vi "UHR-Fleezers Control (host) - Lorentz v4.vi"() -> ()   [LabVIEW 2014] (continued)
                        n1799 = call "Write to pump.vi"("string"="start", "VISA resource name"=w2795) -> ()  [unwired: 1 out]
                      }
                      frame #3 {
                        n1800 = Wait (ms)(milliseconds to wait=u32 500) -> ()  [unwired: 1 out]
                      }
                      frame #4 {
                        n1801 = call "Write to pump.vi"("string"="start", "VISA resource name"=w2799) -> ()  [unwired: 1 out]
                      }
                    }
                  }
                }
              }
              frame True {
                n1802 = case shown="False" w2804 {
                  tunnel: w2805 -> [w2817 w2827]
                  frame False {
                    n1803 = flat-sequence {
                      tunnel: w2817 -> [w2819]
                      frame #0 {
                        n1804 = local write "Flushing P1"(FALSE ("Flushing P1")) -> ()
                        n1805 = Concatenate Strings("stop" ("string"), "\r") -> (w2821:string)
                        n1806 = VISA Write(VISA resource name=w2819, write buffer=w2821) -> ()  [unwired: 1 in, 3 out]
                      }
                      frame #1 {
                        n1807 = property on="Clear Volume P1" class="Bool (strict)"("Val(Sgnl)"=TRUE ("Value (Signaling)")) -> ()  [unwired: 2 in, 2 out]
                      }
                    }
                  }
                  frame True {
                    n1808 = local read "Normal Flow Rate (ul/h) P1"() -> (w2825:dbl)
                    n1809 = Number To Decimal String(number=w2825) -> (decimal integer string=w2831:string)  [unwired: 1 in]
                    n1810 = Concatenate Strings("irate  " ("string"), w2831, " u/h" ("string"), "\r") -> (w2829:string)
                    n1811 = VISA Write(VISA resource name=w2827, write buffer=w2829) -> (VISA resource name out=w2826:refnum<visa-resource-name>)  [unwired: 1 in, 2 out]
                    n1812 = Concatenate Strings("irun" ("string"), "\r") -> (w2833:string)
                    n1813 = VISA Write(VISA resource name=w2826, write buffer=w2833) -> ()  [unwired: 1 in, 3 out]
                  }
                }
                n1814 = local read "Saving..."() -> (w2802:bool)
                n1815 = local read "Save Event Log?"() -> (w2801:bool)
                n1816 = And(x=w2802, y=w2801) -> (x .and. y?=w2803:bool)
                n1817 = case shown="True" w2803 {
                  tunnel: w2804 -> [_ w2815]
                  frame False {
                  }
                  frame True {
                    n1818 = local read "Normal Flow Rate (ul/h) P1"() -> (w2806:dbl)
                    n1819 = Number To Decimal String(number=w2806) -> (decimal integer string=w2807:string)  [unwired: 1 in]
                    n1820 = Concatenate Strings("on, flow rate", w2807) -> (w2809:string)
                    n1821 = Select(t=w2809, s=w2815, f="off") -> (s? t:f=w2811:string)
                    n1822 = local read "log file ref"() -> (w2816:refnum<file>)
                    n1823 = local read "Time (s)"() -> (w2810:dbl)
                    n1824 = Concatenate Strings("pump 1 ", w2811) -> (w2813:string)
                    n1825 = call "write to event log.vi"("log file ref"=w2816, "time"=w2810, "input string"=w2813) -> ()  [unwired: 8 in]
                  }
                }
              }
            }
          }
          frame Enabled {
          }
        }
      }
      event "Shunt 1": Value Change {
        n1826 = event-data() -> ()  [unwired: 7 out]
        n1827 = local read "Visa resource for valves"() -> (w2835:refnum<visa-resource-name>)
        n1828 = call "hamilton_controller.vi"("VISA resource name in"=w2835, "Open?"="Shunt 1", "valve"=enum16{"A", "B", "ALL"}."A", "action"=T53."MOVE VALVE") -> ("error out"=w2837:errorcluster)  [unwired: 6 in, 1 out]
      }
      event "Shunt 2": Value Change {
        n1829 = event-data() -> ()  [unwired: 7 out]
        n1830 = local read "Visa resource for valves"() -> (w2840:refnum<visa-resource-name>)
        n1831 = call "hamilton_controller.vi"("VISA resource name in"=w2840, "Open?"="Shunt 2", "valve"=enum16{"A", "B", "ALL"}."B", "action"=T53."MOVE VALVE") -> ("error out"=w2841:errorcluster)  [unwired: 6 in, 1 out]
      }
      event "Inject Pump 3": Value Change {
        n1832 = event-data() -> ()  [unwired: 7 out]
        n1833 = local read "Use Harvard pumps\nfor beads (else Chemyx)"() -> (w2846:bool)
        n1834 = disable-structure shown="Disabled" {
          disable-tunnel: w2846 -> [w2848 _]
          disable-tunnel: w2845 -> [w2847 _]
          frame Disabled {
            n1835 = case shown="True" w2848 {
              tunnel: "Inject Pump 3" -> [w2852 w2893]
              tunnel: w2847 -> [_ w2894]
              frame False {
                n1836 = local read "Pump write delay (ms)"() -> (w2851:dbl)
                n1837 = case shown="True" w2852 {
                  tunnel: w2851 -> [w2858 w2872]
                  tunnel: "Chemyx Syringe Pump Serial Port" -> [w2855 w2871]
                  frame False {
                    n1838 = flat-sequence {
                      tunnel: w2855 -> [w2859]
                      tunnel: [w2859] -> w2856
                      tunnel: w2858 -> [_]
                      tunnel: [w2862] -> w2857
                      tunnel: w2856 -> [w2862]
                      tunnel: w2857 -> [w2863]
                      tunnel: [w2863] -> w2853
                      tunnel: [w2865] -> w2854
                      tunnel: w2853 -> [w2865]
                      tunnel: w2854 -> [w2867]
                      frame #0 {
                        n1839 = call "Write to pump.vi"("string"="enter pump3", "VISA resource name"=w2859) -> ()  [unwired: 1 out]
                      }
                      frame #1 {
                        n1840 = local read "Pump pause delay (ms)"() -> (w2861:u32)
                        n1841 = Wait (ms)(milliseconds to wait=w2861) -> ()  [unwired: 1 out]
                      }
                      frame #2 {
                        n1842 = call "Write to pump.vi"("string"="stop", "VISA resource name"=w2863) -> ()  [unwired: 1 out]
                      }
                      frame #3 {
                        n1843 = Wait (ms)(milliseconds to wait=u32 0) -> ()  [unwired: 1 out]
                      }
                      frame #4 {
                        n1844 = call "Write to pump.vi"("string"="stop", "VISA resource name"=w2867) -> ()  [unwired: 1 out]
                      }
                    }
                  }
                  frame True {
                    n1845 = flat-sequence {
                      tunnel: w2871 -> [w2881]
                      tunnel: w2872 -> [w2876]
                      tunnel: w2872 -> [w2883]
                      tunnel: w2871 -> [w2884]
                      tunnel: [w2884] -> w2870
                      tunnel: [w2887] -> w2869
                      tunnel: w2870 -> [w2887]
                      tunnel: w2869 -> [w2888]
                      frame #0 {
                        n1846 = local read "All Pump Parameters"() -> (w2875:T10)
                        n1847 = Unbundle By Name(w2875) -> ("Pump 3"=w2882:T57)
                        n1848 = call "Set pump parameters.vi"("Pump write delay (ms)"=w2876, "Volume (uL)"="Ch 3 Inject Volume (uL)", "Rate (uL/h)"="Ch 3 Inject Rate (ul/h)", "Units"=4.0, "Pump #"=3.0, "Pump Parameters In"=w2882, "VISA resource name"=w2881) -> ("Pump Parameters Out"=w2874:T57)  [unwired: 3 in]
                        n1849 = Bundle By Name(cluster=w2875, "Pump 3"=w2874) -> (w2873:T10)
                        n1850 = local write "All Pump Parameters"(w2873) -> ()
                      }
                      frame #1 {
                        n1851 = Wait (ms)(milliseconds to wait=w2883) -> ()  [unwired: 1 out]
                      }
                      frame #2 {
                        n1852 = call "Write to pump.vi"("string"="start", "VISA resource name"=w2884) -> ()  [unwired: 1 out]
                      }
                      frame #3 {
                        n1853 = Wait (ms)(milliseconds to wait=u32 500) -> ()  [unwired: 1 out]
                      }
                      frame #4 {
                        n1854 = call "Write to pump.vi"("string"="start", "VISA resource name"=w2888) -> ()  [unwired: 1 out]
                      }
                    }
                  }
                }
              }
              frame True {
                n1855 = case shown="False" w2893 {
                  tunnel: w2894 -> [w2906 w2913]
                  frame False {
                    n1856 = flat-sequence {
                      tunnel: w2906 -> [w2908]
                      frame #0 {
                        n1857 = local write "Flushing P3"(FALSE ("Flushing P3")) -> ()
                        n1858 = Concatenate Strings("stop" ("string"), "\r") -> (w2910:string)
                        n1859 = VISA Write(VISA resource name=w2908, write buffer=w2910) -> ()  [unwired: 1 in, 3 out]
                      }
                      frame #1 {
                        n1860 = property on="Clear Volume P3" class="Bool (strict)"("Val(Sgnl)"=TRUE ("Value (Signaling)")) -> ()  [unwired: 2 in, 2 out]
                      }
                    }
                  }
                  frame True {
                    n1861 = local read "Normal Flow Rate (ul/h) P3"() -> (w2914:dbl)
                    n1862 = Number To Decimal String(number=w2914) -> (decimal integer string=w2920:string)  [unwired: 1 in]
                    n1863 = Concatenate Strings("irate  " ("string"), w2920, " u/h" ("string"), "\r") -> (w2918:string)
                    n1864 = VISA Write(VISA resource name=w2913, write buffer=w2918) -> (VISA resource name out=w2916:refnum<visa-resource-name>)  [unwired: 1 in, 2 out]
                    n1865 = Concatenate Strings("irun" ("string"), "\r") -> (w2922:string)
                    n1866 = VISA Write(VISA resource name=w2916, write buffer=w2922) -> ()  [unwired: 1 in, 3 out]
                  }
                }
                n1867 = local read "Save Event Log?"() -> (w2891:bool)
                n1868 = local read "Saving..."() -> (w2892:bool)
                n1869 = And(x=w2892, y=w2891) -> (x .and. y?=w2890:bool)
                n1870 = case shown="True" w2890 {
                  tunnel: w2893 -> [_ w2901]
                  frame False {
                  }
                  frame True {
                    n1871 = local read "Normal Flow Rate (ul/h) P3"() -> (w2895:dbl)
                    n1872 = Number To Decimal String(number=w2895) -> (decimal integer string=w2897:string)  [unwired: 1 in]
                    n1873 = Concatenate Strings("on, flow rate", w2897) -> (w2896:string)
                    n1874 = local read "log file ref"() -> (w2900:refnum<file>)
                    n1875 = Select(t=w2896, s=w2901, f="off") -> (s? t:f=w2902:string)
                    n1876 = local read "Time (s)"() -> (w2899:dbl)
                    n1877 = Concatenate Strings("pump 3 ", w2902) -> (w2904:string)
                    n1878 = call "write to event log.vi"("log file ref"=w2900, "time"=w2899, "input string"=w2904) -> ()  [unwired: 8 in]
                  }
                }
              }
            }
          }
          frame Enabled {
          }
        }
      }
      event "Inject Pump 2": Value Change {
        n1879 = event-data() -> ()  [unwired: 7 out]
        n1880 = local read "Pump write delay (ms)"() -> (w2929:dbl)
        n1881 = local read "Chemyx Syringe Pump Serial Port"() -> (w2928:refnum<visa-resource-name>)
        n1882 = flat-sequence {
          tunnel: w2928 -> [w2953]
          tunnel: w2929 -> [w2949]
          tunnel: "Inject Pump 2" -> [_]
          tunnel: w2929 -> [w2955]
          tunnel: w2928 -> [w2956]
          frame #0 {
            n1883 = local read "All Pump Parameters"() -> (w2948:T10)
            n1884 = Multiply(x=60.0, y="Flush Center Ch Rate (ul/m)") -> (x*y=w2945:dbl)
            n1885 = Unbundle By Name(w2948) -> ("Pump 2"=w2954:T57)
            n1886 = call "Set pump parameters.vi"("Pump write delay (ms)"=w2949, "Volume (uL)"="Flush Center Ch Volume (uL)", "Rate (uL/h)"=w2945, "Units"=3.0, "Pump #"=2.0, "Pump Parameters In"=w2954, "VISA resource name"=w2953) -> ("Pump Parameters Out"=w2947:T57)  [unwired: 3 in]
            n1887 = Bundle By Name(cluster=w2948, "Pump 2"=w2947) -> (w2946:T10)
            n1888 = local write "All Pump Parameters"(w2946) -> ()
            n1889 = Add(x="Flush Center Ch Volume (uL)", y="Total Volume\nFlushed (uL)") -> (x+y=w2942:dbl)
            n1890 = local write "Total Volume\nFlushed (uL)"(w2942) -> ()
          }
          frame #1 {
            n1891 = Wait (ms)(milliseconds to wait=w2955) -> ()  [unwired: 1 out]
          }
          frame #2 {
            n1892 = call "Write to pump.vi"("string"="start", "VISA resource name"=w2956) -> ()  [unwired: 1 out]
          }
        }
        n1893 = local read "Save Event Log?"() -> (w2927:bool)
        n1894 = local read "Saving..."() -> (w2926:bool)
        n1895 = And(x=w2927, y=w2926) -> (x .and. y?=w2925:bool)
        n1896 = case shown="True" w2925 {
          tunnel: "Inject Pump 2" -> [_ w2936]
          frame False {
          }
          frame True {
            n1897 = local read "Flow rate (uL/h)"() -> (w2930:dbl)
            n1898 = Number To Decimal String(number=w2930) -> (decimal integer string=w2932:string)  [unwired: 1 in]
            n1899 = Concatenate Strings("on, flow rate", w2932) -> (w2931:string)
            n1900 = Select(t=w2931, s=w2936, f="off") -> (s? t:f=w2940:string)
            n1901 = local read "Time (s)"() -> (w2934:dbl)
            n1902 = local read "log file ref"() -> (w2935:refnum<file>)
            n1903 = Concatenate Strings("pump 2 ", w2940) -> (w2938:string)
            n1904 = call "write to event log.vi"("log file ref"=w2935, "time"=w2934, "input string"=w2938) -> ()  [unwired: 8 in]
          }
        }
      }
      event "Sample Channel\nFlow": Value Change {
        n1905 = event-data() -> ()  [unwired: 7 out]
        n1906 = disable-structure shown="Disabled" {
          disable-tunnel: w2958 -> [w2965 _]
          frame Disabled {
            n1907 = Select(t="irun" ("string"), s="Sample Channel\nFlow", f="stop" ("string")) -> (s? t:f=w2960:string)
            n1908 = Concatenate Strings(w2960, "\r") -> (w2963:string)
            n1909 = VISA Write(VISA resource name=w2965, write buffer=w2963) -> ()  [unwired: 1 in, 3 out]
          }
          frame Enabled {
          }
        }
      }
      event "Start Flow": Value Change {
        n1910 = event-data() -> ()  [unwired: 7 out]
        n1911 = disable-structure shown="Disabled" {
          disable-tunnel: w2966 -> [w2967 _]
          frame Disabled {
            n1912 = local write "Sample Channel\nFlow"(TRUE ("Sample Channel\nFlow")) -> ()
            n1913 = local write "Start Flow"(FALSE ("Start Flow")) -> ()
            n1914 = Concatenate Strings("irun" ("string"), "\r") -> (w2971:string)
            n1915 = VISA Write(VISA resource name=w2967, write buffer=w2971) -> ()  [unwired: 1 in, 3 out]
          }
          frame Enabled {
          }
        }
      }
      event "Stop Flow": Value Change {
        n1916 = event-data() -> ()  [unwired: 7 out]
        n1917 = disable-structure shown="Disabled" {
          disable-tunnel: w2973 -> [w2975 _]
          frame Disabled {
            w2974 = FALSE ("Stop Flow")
            n1918 = local write "Stop Flow"(w2974) -> ()
            n1919 = local write "Sample Channel\nFlow"(w2974) -> ()
            n1920 = Concatenate Strings("stop" ("string"), "\r") -> (w2977:string)
            n1921 = VISA Write(VISA resource name=w2975, write buffer=w2977) -> ()  [unwired: 1 in, 3 out]
          }
          frame Enabled {
          }
        }
      }
      event "Flow rate (uL/h)": Value Change {
        n1922 = event-data() -> ()  [unwired: 7 out]
        n1923 = disable-structure shown="Disabled" {
          disable-tunnel: w2979 -> [w2981 _]
          frame Disabled {
            n1924 = Number To Decimal String(number="Flow rate (uL/h)") -> (decimal integer string=w2985:string)  [unwired: 1 in]
            n1925 = Concatenate Strings("irate  " ("string"), w2985, " u/h" ("string"), "\r") -> (w2984:string)
            n1926 = VISA Write(VISA resource name=w2981, write buffer=w2984) -> ()  [unwired: 1 in, 3 out]
          }
          frame Enabled {
          }
        }
      }
      event "Flush Sample": Value Change {
        n1927 = event-data() -> ()  [unwired: 7 out]
        n1928 = disable-structure shown="Disabled" {
          disable-tunnel: ["Flush Sample" _] -> w2988
          disable-tunnel: w2987 -> [w2994 _]
          frame Disabled {
            n1929 = flat-sequence {
              tunnel: w2994 -> [w3035]
              tunnel: [w3015] -> w2998
              tunnel: [w3011] -> w2997
              tunnel: ["Volume (uL)"] -> w2993
              tunnel: ["Flush rate (uL/m)"] -> w2992
              tunnel: w2998 -> [w3039]
              tunnel: [w3039] -> w2996
              tunnel: w2997 -> [w3038]
              tunnel: w2996 -> [w3044]
              frame #0 {
                # "set paramaters (rate, volume) for flush, clear volume"
                n1930 = Number To Decimal String(number="Flush rate (uL/m)") -> (decimal integer string=w3031:string)  [unwired: 1 in]
                n1931 = Concatenate Strings("irate  " ("string"), w3031, " u/m" ("string"), "\r") -> (w3033:string)
                n1932 = VISA Write(VISA resource name=w3035, write buffer=w3033) -> (VISA resource name out=w3029:refnum<visa-resource-name>)  [unwired: 1 in, 2 out]
                n1933 = Reciprocal(x="Flush rate (uL/m)") -> (1/x=w3014:dbl)
                n1934 = Number To Decimal String(number="Volume (uL)") -> (decimal integer string=w3020:string)  [unwired: 1 in]
                n1935 = Multiply(x="Volume (uL)", y=w3014) -> (x*y=w3013:dbl)
                n1936 = Concatenate Strings("tvolume  " ("string"), w3020, " u" ("string"), "\r") -> (w3018:string)
                n1937 = Multiply(x=w3013, y=60000.0) -> (x*y=w3011:dbl)
                n1938 = VISA Write(VISA resource name=w3029, write buffer=w3018) -> (VISA resource name out=w3017:refnum<visa-resource-name>)  [unwired: 1 in, 2 out]
                n1939 = Concatenate Strings("cvolume" ("string"), "\r") -> (w3016:string)
                n1940 = VISA Write(VISA resource name=w3017, write buffer=w3016) -> (VISA resource name out=w3027:refnum<visa-resource-name>)  [unwired: 1 in, 2 out]
                n1941 = Concatenate Strings("irun" ("string"), "\r") -> (w3025:string)
                n1942 = VISA Write(VISA resource name=w3027, write buffer=w3025) -> (VISA resource name out=w3015:refnum<visa-resource-name>)  [unwired: 1 in, 2 out]
              }
              frame #1 {
                # "Have to wait until\nflow is done to reset\nrate"
                n1943 = Add(x=w3038, y=100.0) -> (x+y=w3037:dbl)
                n1944 = Wait (ms)(milliseconds to wait=w3037) -> ()  [unwired: 1 out]
              }
              frame #2 {
                # "reset flow rate to usual flow rate"
                n1945 = local read "Flow rate (uL/h)"() -> (w3050:dbl)
                n1946 = Number To Decimal String(number=w3050) -> (decimal integer string=w3048:string)  [unwired: 1 in]
                n1947 = Concatenate Strings("irate  " ("string"), w3048, " u/h" ("string"), "\r") -> (w3046:string)
                n1948 = VISA Write(VISA resource name=w3044, write buffer=w3046) -> (VISA resource name out=w3040:refnum<visa-resource-name>)  [unwired: 1 in, 2 out]
                n1949 = Concatenate Strings("cvolume" ("string"), "\r") -> (w3041:string)
                n1950 = VISA Write(VISA resource name=w3040, write buffer=w3041) -> ()  [unwired: 1 in, 3 out]
              }
            }
            n1951 = local read "Save Event Log?"() -> (w2990:bool)
            n1952 = local read "Saving..."() -> (w2989:bool)
            n1953 = And(x=w2990, y=w2989) -> (x .and. y?=w2991:bool)
            n1954 = case shown="True" w2991 {
              tunnel: w2993 -> [_ w3000]
              tunnel: w2992 -> [_ w2999]
              frame False {
              }
              frame True {
                n1955 = Number To Decimal String(number=w3000) -> (decimal integer string=w3004:string)  [unwired: 1 in]
                n1956 = Number To Decimal String(number=w2999) -> (decimal integer string=w3006:string)  [unwired: 1 in]
                n1957 = local read "log file ref"() -> (w3001:refnum<file>)
                n1958 = local read "Time (s)"() -> (w3002:dbl)
                n1959 = Concatenate Strings("pump 2 flushing ", w3004, " uL at ", w3006, " ul/min") -> (w3008:string)
                n1960 = call "write to event log.vi"("log file ref"=w3001, "time"=w3002, "input string"=w3008) -> ()  [unwired: 8 in]
              }
            }
          }
          frame Enabled {
          }
        }
      }
      event "Flush Pump 3": Value Change {
        n1961 = event-data() -> ()  [unwired: 7 out]
        n1962 = disable-structure shown="Disabled" {
          disable-tunnel: ["Flush Pump 3" _] -> w3052
          disable-tunnel: w3051 -> [w3058 _]
          frame Disabled {
            n1963 = flat-sequence {
              tunnel: w3058 -> [w3073]
              tunnel: ["Flush rate (uL/m) P3"] -> w3054
              tunnel: ["Volume (uL) P3"] -> w3053
              frame #0 {
                # "set paramaters (rate, volume) for flush, clear volume"
                n1964 = Number To Decimal String(number="Flush rate (uL/m) P3") -> (decimal integer string=w3093:string)  [unwired: 1 in]
                n1965 = local write "Inject Pump 3"(TRUE ("Inject Pump 3")) -> ()
                n1966 = Concatenate Strings("irate  " ("string"), w3093, " u/m" ("string"), "\r") -> (w3095:string)
                n1967 = VISA Write(VISA resource name=w3073, write buffer=w3095) -> (VISA resource name out=w3091:refnum<visa-resource-name>)  [unwired: 1 in, 2 out]
                n1968 = Reciprocal(x="Flush rate (uL/m) P3") -> (1/x=w3077:dbl)
                n1969 = Number To Decimal String(number="Volume (uL) P3") -> (decimal integer string=w3082:string)  [unwired: 1 in]
                n1970 = Multiply(x="Volume (uL) P3", y=w3077) -> (x*y=w3076:dbl)
                n1971 = Concatenate Strings("tvolume  " ("string"), w3082, " u" ("string"), "\r") -> (w3080:string)
                n1972 = Multiply(x=w3076, y=60.0) -> (x*y=→"HP3 Flush Time (s)":dbl)
                n1973 = VISA Write(VISA resource name=w3091, write buffer=w3080) -> (VISA resource name out=w3079:refnum<visa-resource-name>)  [unwired: 1 in, 2 out]
                n1974 = Concatenate Strings("cvolume" ("string"), "\r") -> (w3078:string)
                n1975 = VISA Write(VISA resource name=w3079, write buffer=w3078) -> (VISA resource name out=w3089:refnum<visa-resource-name>)  [unwired: 1 in, 2 out]
                n1976 = Concatenate Strings("irun" ("string"), "\r") -> (w3087:string)
                n1977 = VISA Write(VISA resource name=w3089, write buffer=w3087) -> ()  [unwired: 1 in, 3 out]
              }
              frame #1 {
                "Flushing P3" <- TRUE ("Flushing P3")
              }
            }
            n1978 = local read "Save Event Log?"() -> (w3056:bool)
            n1979 = local read "Saving..."() -> (w3057:bool)
            n1980 = And(x=w3056, y=w3057) -> (x .and. y?=w3055:bool)
            n1981 = case shown="True" w3055 {
              tunnel: w3054 -> [_ w3061]
              tunnel: w3053 -> [_ w3060]
              frame False {
              }
              frame True {
                n1982 = Number To Decimal String(number=w3060) -> (decimal integer string=w3065:string)  [unwired: 1 in]
                n1983 = Number To Decimal String(number=w3061) -> (decimal integer string=w3067:string)  [unwired: 1 in]
                n1984 = local read "log file ref"() -> (w3062:refnum<file>)
                n1985 = local read "Time (s)"() -> (w3063:dbl)
                n1986 = Concatenate Strings("pump 3 flushing ", w3065, " uL at ", w3067, " ul/min") -> (w3069:string)
                n1987 = call "write to event log.vi"("log file ref"=w3062, "time"=w3063, "input string"=w3069) -> ()  [unwired: 8 in]
              }
            }
          }
          frame Enabled {
          }
        }
      }
      event "Flush Pump 1": Value Change {
        n1988 = event-data() -> ()  [unwired: 7 out]
        n1989 = disable-structure shown="Disabled" {
          disable-tunnel: ["Flush Pump 1" _] -> w3099
          disable-tunnel: w3098 -> [w3105 _]
          frame Disabled {
            n1990 = flat-sequence {
              tunnel: [w3126] -> w3107
              tunnel: w3105 -> [w3121]
              tunnel: ["Volume (uL) P1"] -> w3101
              tunnel: ["Flush rate (uL/m) P1"] -> w3100
              tunnel: w3107 -> [_]
              frame #0 {
                # "set paramaters (rate, volume) for flush, clear volume"
                n1991 = local write "Inject Pump 1"(TRUE ("Inject Pump 1")) -> ()
                n1992 = Number To Decimal String(number="Flush rate (uL/m) P1") -> (decimal integer string=w3142:string)  [unwired: 1 in]
                n1993 = Concatenate Strings("irate  " ("string"), w3142, " u/m" ("string"), "\r") -> (w3144:string)
                n1994 = VISA Write(VISA resource name=w3121, write buffer=w3144) -> (VISA resource name out=w3140:refnum<visa-resource-name>)  [unwired: 1 in, 2 out]
                n1995 = Reciprocal(x="Flush rate (uL/m) P1") -> (1/x=w3125:dbl)
                n1996 = Number To Decimal String(number="Volume (uL) P1") -> (decimal integer string=w3131:string)  [unwired: 1 in]
                n1997 = Multiply(x="Volume (uL) P1", y=w3125) -> (x*y=w3124:dbl)
                n1998 = Concatenate Strings("tvolume  " ("string"), w3131, " u" ("string"), "\r") -> (w3129:string)
                n1999 = Multiply(x=w3124, y=60.0) -> (x*y=→"HP1 Flush Time (s)":dbl)
                n2000 = VISA Write(VISA resource name=w3140, write buffer=w3129) -> (VISA resource name out=w3128:refnum<visa-resource-name>)  [unwired: 1 in, 2 out]
                n2001 = Concatenate Strings("cvolume" ("string"), "\r") -> (w3127:string)
                n2002 = VISA Write(VISA resource name=w3128, write buffer=w3127) -> (VISA resource name out=w3138:refnum<visa-resource-name>)  [unwired: 1 in, 2 out]
                n2003 = Concatenate Strings("irun" ("string"), "\r") -> (w3136:string)
                n2004 = VISA Write(VISA resource name=w3138, write buffer=w3136) -> (VISA resource name out=w3126:refnum<visa-resource-name>)  [unwired: 1 in, 2 out]
              }
              frame #1 {
                "Flushing P1" <- TRUE ("Flushing P3")
              }
            }
            n2005 = local read "Saving..."() -> (w3102:bool)
            n2006 = local read "Save Event Log?"() -> (w3103:bool)
            n2007 = And(x=w3103, y=w3102) -> (x .and. y?=w3104:bool)
            n2008 = case shown="True" w3104 {
              tunnel: w3101 -> [_ w3110]
              tunnel: w3100 -> [_ w3109]
              frame False {
              }
              frame True {
                n2009 = Number To Decimal String(number=w3110) -> (decimal integer string=w3114:string)  [unwired: 1 in]
                n2010 = Number To Decimal String(number=w3109) -> (decimal integer string=w3112:string)  [unwired: 1 in]
                n2011 = local read "log file ref"() -> (w3116:refnum<file>)
                n2012 = local read "Time (s)"() -> (w3117:dbl)
                n2013 = Concatenate Strings("pump 1 flushing ", w3114, " uL at ", w3112, " ul/min") -> (w3108:string)
                n2014 = call "write to event log.vi"("log file ref"=w3116, "time"=w3117, "input string"=w3108) -> ()  [unwired: 8 in]
              }
            }
          }
          frame Enabled {
          }
        }
      }
      event "Clear Volume": Value Change {
        n2015 = event-data() -> ()  [unwired: 7 out]
        n2016 = disable-structure shown="Disabled" {
          disable-tunnel: ["Clear Volume" _] -> w3148
          disable-tunnel: w3147 -> [w3149 _]
          frame Disabled {
            n2017 = Concatenate Strings("cvolume" ("string"), "\r") -> (w3150:string)
            n2018 = VISA Write(VISA resource name=w3149, write buffer=w3150) -> ()  [unwired: 1 in, 3 out]
          }
          frame Enabled {
          }
        }
      }
      event "Clear Volume P3": Value Change {
        n2019 = event-data() -> ()  [unwired: 7 out]
        n2020 = disable-structure shown="Disabled" {
          disable-tunnel: w3154 -> [w3156 _]
          frame Disabled {
            n2021 = Concatenate Strings("cvolume" ("string"), "\r") -> (w3157:string)
            n2022 = VISA Write(VISA resource name=w3156, write buffer=w3157) -> ()  [unwired: 1 in, 3 out]
            n2023 = local write "Clear Volume P3"(FALSE ("Clear Volume P3")) -> ()
          }
          frame Enabled {
          }
        }
      }
      event "Clear Volume P1": Value Change {
        n2024 = event-data() -> ()  [unwired: 7 out]
        n2025 = disable-structure shown="Disabled" {
          disable-tunnel: w3160 -> [w3162 _]
          frame Disabled {
            n2026 = Concatenate Strings("cvolume" ("string"), "\r") -> (w3163:string)
            n2027 = local write "Clear Volume P1"(FALSE ("Clear Volume P1")) -> ()
            n2028 = VISA Write(VISA resource name=w3162, write buffer=w3163) -> ()  [unwired: 1 in, 3 out]
          }
          frame Enabled {
          }
        }
      }
      event "Display On P3": Value Change {
        n2029 = event-data() -> ()  [unwired: 7 out]
        n2030 = disable-structure shown="Disabled" {
          disable-tunnel: w3166 -> [w3167 _]
          frame Disabled {
            n2031 = Select(t="dim 100", s="Display On P3", f="dim 0") -> (s? t:f=w3170:string)
            n2032 = Concatenate Strings(w3170, "\r") -> (w3172:string)
            n2033 = VISA Write(VISA resource name=w3167, write buffer=w3172) -> ()  [unwired: 1 in, 3 out]
          }
          frame Enabled {
          }
        }
      }
      event "Display On P1": Value Change {
        n2034 = event-data() -> ()  [unwired: 7 out]
        n2035 = disable-structure shown="Disabled" {
          disable-tunnel: w3174 -> [w3175 _]
          frame Disabled {
            n2036 = Select(t="dim 100", s="Display On P1", f="dim 0") -> (s? t:f=w3178:string)
            n2037 = Concatenate Strings(w3178, "\r") -> (w3180:string)
            n2038 = VISA Write(VISA resource name=w3175, write buffer=w3180) -> ()  [unwired: 1 in, 3 out]
          }
          frame Enabled {
          }
        }
      }
      event "Retract Pump 3": Value Change {
        n2039 = event-data() -> ()  [unwired: 7 out]
        n2040 = disable-structure shown="Disabled" {
          disable-tunnel: w3182 -> [w3183 _]
          frame Disabled {
            n2041 = local write "Retract Pump 3"(FALSE ("Retract Pump 3")) -> ()
            n2042 = case shown="True" "Retract Pump 3" {
              tunnel: w3183 -> [_ w3186]
              frame False {
              }
              frame True {
                n2043 = Number To Decimal String(number="Retract Rate (uL/m)") -> (decimal integer string=w3204:string)  [unwired: 1 in]
                n2044 = Concatenate Strings("wrate  " ("string"), w3204, " u/m" ("string"), "\r") -> (w3206:string)
                n2045 = VISA Write(VISA resource name=w3186, write buffer=w3206) -> (VISA resource name out=w3197:refnum<visa-resource-name>)  [unwired: 1 in, 2 out]
                n2046 = Number To Decimal String(number="Retract Vol 3 (uL)") -> (decimal integer string=w3199:string)  [unwired: 1 in]
                n2047 = Concatenate Strings("tvolume  " ("string"), w3199, " u" ("string"), "\r") -> (w3196:string)
                n2048 = VISA Write(VISA resource name=w3197, write buffer=w3196) -> (VISA resource name out=w3192:refnum<visa-resource-name>)  [unwired: 1 in, 2 out]
                n2049 = Concatenate Strings("cvolume" ("string"), "\r") -> (w3193:string)
                n2050 = VISA Write(VISA resource name=w3192, write buffer=w3193) -> (VISA resource name out=w3187:refnum<visa-resource-name>)  [unwired: 1 in, 2 out]
                n2051 = Concatenate Strings("wrun" ("string"), "\r") -> (w3188:string)
                n2052 = VISA Write(VISA resource name=w3187, write buffer=w3188) -> ()  [unwired: 1 in, 3 out]
              }
            }
          }
          frame Enabled {
          }
        }
      }
      event "Retract Pump 1": Value Change {
        n2053 = event-data() -> ()  [unwired: 7 out]
        n2054 = disable-structure shown="Disabled" {
          disable-tunnel: w3208 -> [w3209 _]
          frame Disabled {
            n2055 = local write "Retract Pump 1"(FALSE ("Retract Pump 1")) -> ()
            n2056 = case shown="True" "Retract Pump 1" {
              tunnel: w3209 -> [_ w3214]
              frame False {
              }
              frame True {
                n2057 = local read "Retract Rate (uL/m)"() -> (w3212:dbl)
                n2058 = Number To Decimal String(number=w3212) -> (decimal integer string=w3230:string)  [unwired: 1 in]
                n2059 = Concatenate Strings("wrate  " ("string"), w3230, " u/m" ("string"), "\r") -> (w3232:string)
                n2060 = VISA Write(VISA resource name=w3214, write buffer=w3232) -> (VISA resource name out=w3224:refnum<visa-resource-name>)  [unwired: 1 in, 2 out]
                n2061 = Number To Decimal String(number="Retract Vol 1 (uL)") -> (decimal integer string=w3226:string)  [unwired: 1 in]
                n2062 = Concatenate Strings("tvolume  " ("string"), w3226, " u" ("string"), "\r") -> (w3223:string)
                n2063 = VISA Write(VISA resource name=w3224, write buffer=w3223) -> (VISA resource name out=w3220:refnum<visa-resource-name>)  [unwired: 1 in, 2 out]
                n2064 = Concatenate Strings("cvolume" ("string"), "\r") -> (w3221:string)
                n2065 = VISA Write(VISA resource name=w3220, write buffer=w3221) -> (VISA resource name out=w3215:refnum<visa-resource-name>)  [unwired: 1 in, 2 out]
                n2066 = Concatenate Strings("wrun" ("string"), "\r") -> (w3216:string)
                n2067 = VISA Write(VISA resource name=w3215, write buffer=w3216) -> ()  [unwired: 1 in, 3 out]
              }
            }
          }
          frame Enabled {
          }
        }
      }
      event "Flip Green Filter": Value Change {
        n2068 = event-data() -> ()  [unwired: 7 out]
        n2069 = Not(x="Flip Green Filter") -> (.not. x?=w3235:bool)
        n2070 = local write "Flip Green Filter"(w3235) -> ()
        n2071 = flat-sequence {
          tunnel: [w3244] -> w3240
          tunnel: [w3243] -> w3239
          tunnel: w3234 -> [w3242]
          tunnel: [w3247] -> w3238
          tunnel: w3240 -> [w3247]
          tunnel: [w3246] -> w3237
          tunnel: w3239 -> [w3246]
          tunnel: w3238 -> [w3251]
          tunnel: w3237 -> [w3250]
          tunnel: [w3249] -> w3241
          frame #0 {
            n2072 = xnode "Read/Write Control"("FPGA VI Reference In"=w3242, "Green Filter Flipper"=TRUE) -> ("FPGA VI Reference Out"=w3244:T50, "error out"=w3243:errorcluster)  [unwired: 1 in]
          }
          frame #1 {
            n2073 = Wait (ms)(milliseconds to wait=u32 100) -> ()  [unwired: 1 out]
          }
          frame #2 {
            n2074 = xnode "Read/Write Control"("FPGA VI Reference In"=w3251, "error in"=w3250, "Green Filter Flipper"=FALSE) -> ("error out"=w3249:errorcluster)  [unwired: 1 out]
          }
        }
      }
      event "Pump 1 contents", "Pump 3 contents": Value Change {
        n2075 = event-data() -> ()  [unwired: 7 out]
        n2076 = local read "Pump 1 contents"() -> (→"Pump 1 cont disp":string)
        n2077 = local read "Pump 3 contents"() -> (→"Pump 3 cont disp":string)
      }
      event "Reset Trap Pos. FB": Value Change {
        n2078 = event-data() -> ()  [unwired: 7 out]
        n2079 = xnode "Read/Write Control"("FPGA VI Reference In"=w3255, "Trap Pos. FB Reset"="Reset Trap Pos. FB") -> ()  [unwired: 1 in, 2 out]
      }
      event "Rem fb disp offset": Value Change {
        n2080 = event-data() -> ()  [unwired: 7 out]
        n2081 = local write "Rem fb disp offset"(FALSE ("Rem fb disp offset")) -> ()
        n2082 = local read "Mean Trap Positions (nm)"() -> (w3258:T5)
        n2083 = local read "FB Trap Pos Offset"() -> (w3260:dbl)
        n2084 = Unbundle By Name(w3258) -> ("T1 X"=w3257:dbl)
        n2085 = Subtract(x=w3260, y=w3257) -> (x-y=w3259:dbl)
        n2086 = local write "FB Trap Pos Offset"(w3259) -> ()
      }
      event "Threshold (nm)": Value Change {
        n2087 = event-data() -> ()  [unwired: 7 out]
        n2088 = flat-sequence {
          tunnel: [w3265] -> w3263
          tunnel: w3262 -> [w3264]
          tunnel: w3263 -> [w3276]
          frame #0 {
            n2089 = xnode "Read/Write Control"("FPGA VI Reference In"=w3264) -> ("FPGA VI Reference Out"=w3268:T50, "error out"=w3267:errorcluster, "FPGA TTrig Thresh"=w3269:i64)  [unwired: 1 in]
            n2090 = local read "Threshold stored (nm)"() -> (w3275:dbl)
            n2091 = local read "Threshold (nm)"() -> (w3265:dbl)
            n2092 = local read "AOM X Cal (nm/MHz)"() -> (w3273:dbl)
            n2093 = Subtract(x=w3265, y=w3275) -> (x-y=w3274:dbl)
            n2094 = Divide(x=w3274, y=w3273) -> (x/y=w3271:dbl)
            n2095 = call "IR AOM freq to word.vi"("Frequency In (MHz)"=w3271) -> ("Frequency Word Out (double)"=w3272:dbl)
            n2096 = To Quad Integer(1:w3272) -> (0:w3270:i64)
            n2097 = Add(x=w3269, y=w3270) -> (x+y=w3266:i64)
            n2098 = xnode "Read/Write Control"("FPGA VI Reference In"=w3268, "error in"=w3267, "FPGA TTrig Thresh"=w3266) -> ()  [unwired: 2 out]
          }
          frame #1 {
            "Threshold stored (nm)" <- w3276
          }
        }
      }
      event "FB Trig Integrate": Value Change {
        n2099 = event-data() -> ()  [unwired: 7 out]
        n2100 = local read "FB Trig Integrate"() -> (w3279:u32)
        n2101 = xnode "Read/Write Control"("FPGA VI Reference In"=w3277, "FB Trig Integrate"=w3279) -> ("error out"=w3278:errorcluster)  [unwired: 1 in, 1 out]
      }
      event "11": Value Change {
        n2102 = event-data() -> ()  [unwired: 7 out]
        n2103 = local read "11"() -> (w3280:bool)
        n2104 = case shown="True" w3280 {
          frame False {
          }
          frame True {
            n2105 = local read "Messages"() -> (w3282:string)
            n2106 = call "Update messages.vi"("Message to add"="You kicked it up to 11!", "Old message string"=w3282) -> ("New message string"=w3283:string)
            n2107 = call <vilib>:"Beep.vi"() -> ()  [unwired: 12 in]
            n2108 = local write "Messages"(w3283) -> ()
          }
        }
      }
      event "Trap Pos. FB ON": Value Change {
        w3290 = 6.0  # clock mult.
        w3289 = 49152000.0  # TCXO frequ.
        n2109 = event-data() -> ()  [unwired: 7 out]
        n2110 = xnode "Read/Write Control"("FPGA VI Reference In"=w3284) -> ("FPGA VI Reference Out"=w3286:T50, "BD1 Frequency Out 1"=w3287:u64)  [unwired: 1 in, 1 out]
        n2111 = To Double Precision Float(number=w3287) -> (double precision float=w3291:dbl)
        n2112 = Multiply(x=w3289, y=w3290) -> (x*y=w3292:dbl)
        n2113 = Multiply(x=w3291, y=w3292) -> (x*y=w3293:dbl)
        n2114 = Scale By Power Of 2(n=-48, x=w3293) -> (x*2^n=w3295:dbl)
        n2115 = Divide(x=w3295, y=1000000.0) -> (x/y=w3288:dbl)
        n2116 = flat-sequence {
          tunnel: w3286 -> [w3301]
          tunnel: [w3300] -> w3297
          tunnel: "Trap Pos. FB ON" -> [w3299]
          tunnel: w3287 -> [w3298]
          tunnel: w3297 -> [w3307]
          tunnel: "Trap Pos. FB ON" -> [w3306]
          tunnel: w3288 -> [w3309]
          tunnel: "Trap Pos. FB ON" -> [w3308]
          frame #0 {
            n2117 = case shown="False" w3299 {
              tunnel: w3301 -> [w3303 w3305]
              tunnel: [w3304 w3305] -> w3300
              tunnel: w3298 -> [w3302 _]
              frame False {
                n2118 = xnode "Read/Write Control"("FPGA VI Reference In"=w3303, "BD 1 Frequency 1"=w3302) -> ("FPGA VI Reference Out"=w3304:T50)  [unwired: 1 in, 1 out]
              }
              frame True {
              }
            }
          }
          frame #1 {
            n2119 = xnode "Read/Write Control"("FPGA VI Reference In"=w3307, "Force feedback"=w3306) -> ()  [unwired: 1 in, 2 out]
          }
          frame #2 {
            n2120 = case shown="False" w3308 {
              tunnel: w3309 -> [w3310 _]
              frame False {
                n2121 = property on="BD 1 Frequency 1 (MHz)" class="DigNum (strict)"("Val(Sgnl)"=w3310) -> ()  [unwired: 2 in, 2 out]
              }
              frame True {
              }
            }
          }
        }
      }
      event "Remove Action Offset": Value Change {
        n2122 = event-data() -> ()  [unwired: 7 out]
        n2123 = local write "Remove Action Offset"(FALSE ("Remove Action Offset")) -> ()
        n2124 = local read "Trap Pos. FB Mult Factor"() -> (w3316:i64)
        n2125 = local read "Trap Pos FB Action"() -> (w3314:i64)
        n2126 = local read "Trap Pos. FB Offset Factor"() -> (w3312:i64)
        n2127 = Multiply(x=w3316, y=w3314) -> (x*y=w3315:i64)
        n2128 = Add(x=w3315, y=w3312) -> (x+y=w3313:i64)
        n2129 = local write "Trap Pos. FB Offset Factor"(w3313) -> ()
        n2130 = xnode "Read/Write Control"("FPGA VI Reference In"=w3311, "Trap Pos. FB Offset Factor"=w3313) -> ()  [unwired: 1 in, 2 out]
      }
      event "Remove Unwinding Offset": Value Change {
        n2131 = event-data() -> ()  [unwired: 7 out]
        n2132 = local write "Remove Unwinding Offset"(FALSE ("Remove Action Offset")) -> ()
        n2133 = local read "Trap Pos. FB Mult Factor"() -> (w3330:i64)
        n2134 = local read "Trap Pos FB Action"() -> (w3328:i64)
        n2135 = local read "Trap Pos. FB Offset Factor"() -> (w3327:i64)
        n2136 = Multiply(x=w3330, y=w3328) -> (x*y=w3329:i64)
        n2137 = local read "Trap Pos. FB Mult Factor"() -> (w3326:i64)
        n2138 = Add(x=w3329, y=w3327) -> (x+y=w3320:i64)
        n2139 = Multiply(x=32768, y="factor") -> (x*y=w3323:dbl)
        n2140 = Multiply(x=w3323, y=w3326) -> (x*y=w3325:dbl)
        n2141 = Subtract(x=w3320, y=w3325) -> (x-y=w3324:dbl)
        n2142 = To Quad Integer(1:w3324) -> (0:w3319:i64)
        n2143 = xnode "Read/Write Control"("FPGA VI Reference In"=w3318, "Trap Pos. FB Offset Factor"=w3319) -> ()  [unwired: 1 in, 2 out]
        n2144 = local write "Trap Pos. FB Offset Factor"(w3319) -> ()
      }
      event "Trap Pos. FB Range", "Trap Pos. FB Gains", "Trap Pos. FB Mult Factor", "Trap Pos. FB Offset Factor", "Trap Pos FB Negate Action", "Trap Pos FB Monitor\nT1 or T2", "Differential FB?", "Negate Diff?": Value Change {
        n2145 = event-data() -> ()  [unwired: 7 out]
        n2146 = local read "Negate Diff?"() -> (w3335:bool)
        n2147 = xnode "Read/Write Control"("FPGA VI Reference In"=w3334, "Trap Pos. FB Gains"="Trap Pos. FB Gains", "Trap pos. FB Range"="Trap Pos. FB Range", "Trap Pos. FB Mult Factor"="Trap Pos. FB Mult Factor", "Trap Pos. FB Offset Factor"="Trap Pos. FB Offset Factor", "Trap Pos FB Negate Action"="Trap Pos FB Negate Action", "Trap Pos FB Monitor T1 or T2"="Trap Pos FB Monitor\nT1 or T2", "AI1 X Scale"="Trap Pos. AI1 X Pre-scale", "Negate Diff?"=w3335, "Diff FB Measurement?"="Differential FB?") -> ()  [unwired: 1 in, 2 out]
      }
      event "Trap Pos FB SP", "Trap Pos FB SP 2", "Use SP 2": Value Change {
        n2148 = event-data() -> ()  [unwired: 7 out]
        n2149 = Select(t="Trap Pos FB SP 2", s="Use SP 2", f="Trap Pos FB SP") -> (s? t:f=w3343:fxp<+/-,16,1>)
        n2150 = xnode "Read/Write Control"("FPGA VI Reference In"=w3342, "Trap Pos. FB SP"=w3343) -> ()  [unwired: 1 in, 2 out]
      }
      event "Offset SP2 from SP1": Value Change {
        n2151 = event-data() -> ()  [unwired: 7 out]
        n2152 = local read "Trap Pos FB SP"() -> (w3349:fxp<+/-,16,1>)
        n2153 = Add(x=w3349, y="SP2 Offset") -> (x+y=w3347:fxp<+/-,16,1>)
        n2154 = property on="Trap Pos FB SP 2" class="DigNum (strict)"("Val(Sgnl)"=w3347) -> ()  [unwired: 2 in, 2 out]
        n2155 = local write "Offset SP2 from SP1"(FALSE ("Offset SP2 from SP1")) -> ()
      }
      event "Set Reading to\nSetpoint": Value Change {
        # "This is the actual PID input signal"
        n2156 = event-data() -> ()  [unwired: 7 out]
        n2157 = local write "Set Reading to\nSetpoint"(FALSE ("Set SP to Reading")) -> ()
        n2158 = xnode "Read/Write Control"("FPGA VI Reference In"=w3353) -> ("FPGA VI Reference Out"=w3356:T50, "error out"=w3355:errorcluster, "Trap Pos FB Int-Norm Signal"=w3354:fxp<+/-,16,1>, "BD1 Frequency Out 1"=w3352:u64)  [unwired: 1 in]
        n2159 = local read "Differential FB?"() -> (w3357:bool)
        n2160 = case shown="False" w3357 {
          tunnel: [w3386 w3393] -> w3351
          tunnel: w3354 -> [w3384 w3393]
          frame False {
            n2161 = local read "Trap Pos FB Monitor\nT1 or T2"() -> (w3389:bool)
            n2162 = local read "Trap X AI1 (DMA)"() -> (w3392:T19)
            n2163 = Unbundle By Name(w3392) -> ("Set 1"=w3391:fxp<+/-,16,1>, "Set 2"=w3390:fxp<+/-,16,1>)
            n2164 = Select(t=w3391, s=w3389, f=w3390) -> (s? t:f=w3388:fxp<+/-,16,1>)
            n2165 = Not(x="Set SP Using...") -> (.not. x?=w3385:bool)
            n2166 = Select(t=w3384, s=w3385, f=w3388) -> (s? t:f=w3386:fxp<+/-,16,1>)
          }
          frame True {
          }
        }
        n2167 = disable-structure shown="Disabled" {
          disable-tunnel: _ -> [w3362 _]
          disable-tunnel: w3352 -> [w3361 _]
          disable-tunnel: w3351 -> [w3360 _]
          frame Disabled {
            n2168 = case shown="True" w3362 {
              tunnel: [w3363 w3365] -> w3359
              tunnel: w3360 -> [w3363 w3364]
              tunnel: w3361 -> [_ w3383]
              frame False {
              }
              frame True {
                w3381 = 6.0  # clock mult.
                w3382 = 49152000.0  # TCXO frequ.
                # "Added by Ronen - for the real time\nchange of the setpoint to accomodate \nchanges in the offset."
                n2169 = To Double Precision Float(number=w3383) -> (double precision float=w3380:dbl)
                n2170 = local read "BD 1 Frequency 2 (MHz)"() -> (w3373:dbl)
                n2171 = Multiply(x=w3382, y=w3381) -> (x*y=w3379:dbl)
                n2172 = Multiply(x=w3380, y=w3379) -> (x*y=w3378:dbl)
                n2173 = local read "Offset file step size"() -> (w3371:dbl)
                n2174 = Scale By Power Of 2(n=-48, x=w3378) -> (x*2^n=w3376:dbl)
                n2175 = Divide(x=w3376, y=1000000.0) -> (x/y=w3374:dbl)
                n2176 = Subtract(x=w3373, y=w3374) -> (x-y=w3372:dbl)
                n2177 = Divide(x=w3372, y=w3371) -> (x/y=w3370:dbl)
                n2178 = local read item#-1() -> (w3368)
                n2179 = To Long Integer(number=w3370) -> (32bit integer=w3369:i32)
                n2180 = Index Array(array=w3368, index=w3369) -> (element=w3367)
                n2181 = To Fixed-Point(number=w3367) -> (fixed-point=w3366:fxp<+/-,16,1>)  [unwired: 1 in]
                n2182 = Add(x=w3364, y=w3366) -> (x+y=w3365:fxp<+/-,17,2>)
              }
            }
            "Offset corrected setpoint" <- w3359
          }
          frame Enabled {
          }
        }
        n2183 = local write "Trap Pos FB SP"(w3351) -> ()
        n2184 = xnode "Read/Write Control"("FPGA VI Reference In"=w3356, "error in"=w3355, "Trap Pos. FB SP"=w3351) -> ()  [unwired: 2 out]
      }
      event "Trap Pos. FB Out Scale 2^n": Value Change {
        n2185 = event-data() -> ()  [unwired: 7 out]
        n2186 = Scale By Power Of 2(n="Trap Pos. FB Out Scale 2^n", x=ext 1.0) -> (x*2^n=w3394:ext)
        n2187 = property on="Trap Pos. FB Mult Factor" class="DigNum (strict)"("Val(Sgnl)"=w3394) -> ()  [unwired: 2 in, 2 out]
      }
      event "Trap Pos FB Int Count": Value Change {
        n2188 = event-data() -> ()  [unwired: 7 out]
        n2189 = xnode "Read/Write Control"("FPGA VI Reference In"=w3397, "Trap Pos FB Int Count"="Trap Pos FB Int Count") -> ()  [unwired: 1 in, 2 out]
      }
      event "Display Saved Data": Value Change {
        n2190 = event-data() -> ()  [unwired: 7 out]
        n2191 = case shown="\"Amp Current\"" "Display Saved Data" {
          frame "Bead Seperation", Default {
            n2192 = property on="Amp current" class="WFGraph (strict)"("Visible"=FALSE) -> ()  [unwired: 2 in, 2 out]
            n2193 = property on="Trap Delta Graph" class="WFGraph (strict)"("Visible"=TRUE) -> ()  [unwired: 2 in, 2 out]
            n2194 = property on="Saved trap pos" class="WFGraph (strict)"("Visible"=FALSE) -> ()  [unwired: 2 in, 2 out]
          }
          frame "Amp Current" {
            n2195 = property on="Saved trap pos" class="WFGraph (strict)"("Visible"=FALSE) -> ()  [unwired: 2 in, 2 out]
            n2196 = property on="Trap Delta Graph" class="WFGraph (strict)"("Visible"=FALSE) -> ()  [unwired: 2 in, 2 out]
            n2197 = property on="Amp current" class="WFGraph (strict)"("Visible"=TRUE) -> ()  [unwired: 2 in, 2 out]
          }
          frame "Trap Position" {
            n2198 = property on="Saved trap pos" class="WFGraph (strict)"("Visible"=TRUE) -> ()  [unwired: 2 in, 2 out]
            n2199 = property on="Trap Delta Graph" class="WFGraph (strict)"("Visible"=FALSE) -> ()  [unwired: 2 in, 2 out]
            n2200 = property on="Amp current" class="WFGraph (strict)"("Visible"=FALSE) -> ()  [unwired: 2 in, 2 out]
          }
        }
      }
      event "Calibration": Value Change {
        n2201 = event-data() -> ()  [unwired: 7 out]
        n2202 = local read "X or Y?"() -> (w3425:bool)
        n2203 = local read "Calibration"() -> (w3422:u16)
        n2204 = Select(t="X" ("Label.Text"), s=w3425, f="Y" ("Label.Text")) -> (s? t:f=w3419:string)
        n2205 = case shown="0, Default" w3422 {
          tunnel: ["Position (V)" ("Label.Text") "Position (nm)" ("Label.Text") "Force (pN)" ("Label.Text")] -> w3416
          tunnel: [" (V)" ("Label.Text") " (nm)" ("Label.Text") " (pN)" ("Label.Text")] -> w3413
          frame 0, Default {
          }
          frame 1 {
          }
          frame 2 {
          }
        }
        n2206 = Concatenate Strings("T1 " ("Label.Text"), w3419) -> (w3415:string)
        n2207 = Concatenate Strings("T2 " ("Label.Text"), w3419) -> (w3414:string)
        n2208 = property on="Force" class="WFChart (strict)"("YScale.NameLbl.Text"=w3416) -> ()  [unwired: 2 in, 2 out]
        n2209 = Concatenate Strings("Mean" ("Label.Text"), w3413) -> (w3412:string)
        n2210 = Concatenate Strings(w3415, w3413) -> (w3411:string)
        n2211 = Concatenate Strings(w3414, w3413) -> (w3410:string)
        n2212 = Concatenate Strings("Difference" ("Label.Text"), w3413) -> (w3409:string)
        n2213 = property on="Mean" class="DigNum (strict)"("Caption.Text"=w3412) -> ()  [unwired: 2 in, 2 out]
        n2214 = property on="T1 X" class="DigNum (strict)"("Caption.Text"=w3411) -> ()  [unwired: 2 in, 2 out]
        n2215 = property on="T2 X" class="DigNum (strict)"("Caption.Text"=w3410) -> ()  [unwired: 2 in, 2 out]
        n2216 = property on="Difference" class="DigNum (strict)"("Caption.Text"=w3409) -> ()  [unwired: 2 in, 2 out]
      }
      event "Base N trap periods", "Period scale factor", "Trap osc amp (MHz)", "Cal sets to save", "# Samples/trap", "Total Counts (ticks)": Value Change {
        w3432 = 1.0
        w3438 = u32 0 ("y")
        # "scales 0 to 2pi"
        # "Create vector of trap offset (oscillation) values."
        # "Compute oscillation period as a multiple of the trap period. Should also fit nicely as a factor of the DMA period.\nCompare ticks for accurate commensurability check."
        # "Oscillation frequency needs to be commensurate\nwith the data save time."
        # "Be commensurate with total save time/100 (or so). That way you are guaranteed you can average spectra at least 100x."
        n2217 = event-data() -> ()  [unwired: 7 out]
        n2218 = local read "Total Counts (ticks)"() -> (w3454:u16)
        n2219 = To Unsigned Long Integer(number=w3454) -> (unsigned 32bit integer=w3464:u32)
        n2220 = Multiply "Base osc period (ticks)"(x=w3464, y="Base N trap periods") -> (x*y=w3455:u32)
        n2221 = local read "# Samples/trap"() -> (w3459:u32)
        n2222 = Multiply "Scaled osc period (ticks)"(x=w3455, y="Period scale factor") -> (x*y=w3456:dbl)
